vi "3 OCU.vi"(11 "MissionQueue":refnum<class "MissionQueue.lvclass">) -> ()   [LabVIEW 2011]
uses:
  2-RIO/2 Typedefs/setpoints to boat.ctl
  2-RIO/2 Typedefs/sail setpt.ctl
  2-RIO/2 Typedefs/rudder angle.ctl
  2-RIO/2 Typedefs/Velocity.ctl
  2-RIO/2 Typedefs/apparent wind direction.ctl
  2-RIO/2 Typedefs/apparent wind speed.ctl
  2-RIO/2 Typedefs/apparent wind.ctl
  2-RIO/2 Typedefs/heading.ctl
  2-RIO/2 Typedefs/UTM Location.ctl
  2-RIO/2 Typedefs/Which Boat.ctl
  2-RIO/2 Typedefs/generalized sensor status.ctl
  2-RIO/2 Typedefs/indicator LED.ctl
  2-RIO/2 Typedefs/generalized actuator status.ctl
  Classes/Missions/MissionQueue/MissionQueue.lvclass
  2x3-RIO-OCU Comm/2x3 Typedefs/missionTypes.ctl
  2-RIO/2 Typedefs/manual override.ctl
  2-RIO/2 Globals/2 Global.vi
  Classes/Missions/Drive/Drive.lvclass
panel:
  out "Override Rudder Angle":dbl(slide) scale=-30.0..30.0
  out "Override Sail Value":dbl(slide) scale=0.0..1.0
  in  "OVERRIDE?":bool
  in  "OCU Tab Control":T1(tab)
  out "Connected":bool
  in  "Connect":bool
  out "Rudder Actuator Status":T2
  out "Sail Actuator Status":T2
  out "Wind Sensor Status":T4
  out "Location Sensor Status":T4
  out "Direction Sensor Status":T4
  in  "Add Mission":bool
  in  "Load":bool
  in  "Load Mission":path
  in  "Mission Types":T5
  in  "Desired UTM\nLocation (Drive)":T6 caption="Desired UTM Location"
  in  "Distance \nThreshold (Drive)":dbl caption="Distance Threshold"
  in  "Globals":T7(tab)
  out "Which Boat Am I?":T8 items=["Small RC", "Large RC", "Final Boat", "Simulator"]
  in  "Battery Voltage":dbl
  out "Robot\nHeading":T9 format="%05.1f"
  out "Robot UTM Location":T6
  out "Robot Velocity":T10
  out "Overview Image":T11(plugin-control)
  out "Absolute Wind":T10
  out "Apparent Wind\nDirection":T12
  out "Apparent Wind\nSpeed":T13
  out "Apparent Wind":T14
  out "Current Destination":T6
  out "Setpoints to boat":T15
  out "Sail Position":T16
  out "Rudder Angle":T17
  # "Manual Overide Control"
  # "Full Out = RIGHT"
  # "Out = UP"
  # "In = DOWN"
  # "Full In = LEFT"
  # "PORT"
  # "STARB"
  # "A"
  # "G"
  # "S"
  # "<--"
  # "D"
  # "-->"
  # "F"
  # "should be a map here that you can clique on"
  # "logging..."
  # "As Measured"
  # "From Planning Functions"
  # "Path Planning"
  # "(this is not a cluster because subitems\nare generated in parallel code)"
  # "Mission Definition Stuff Goes HERE"
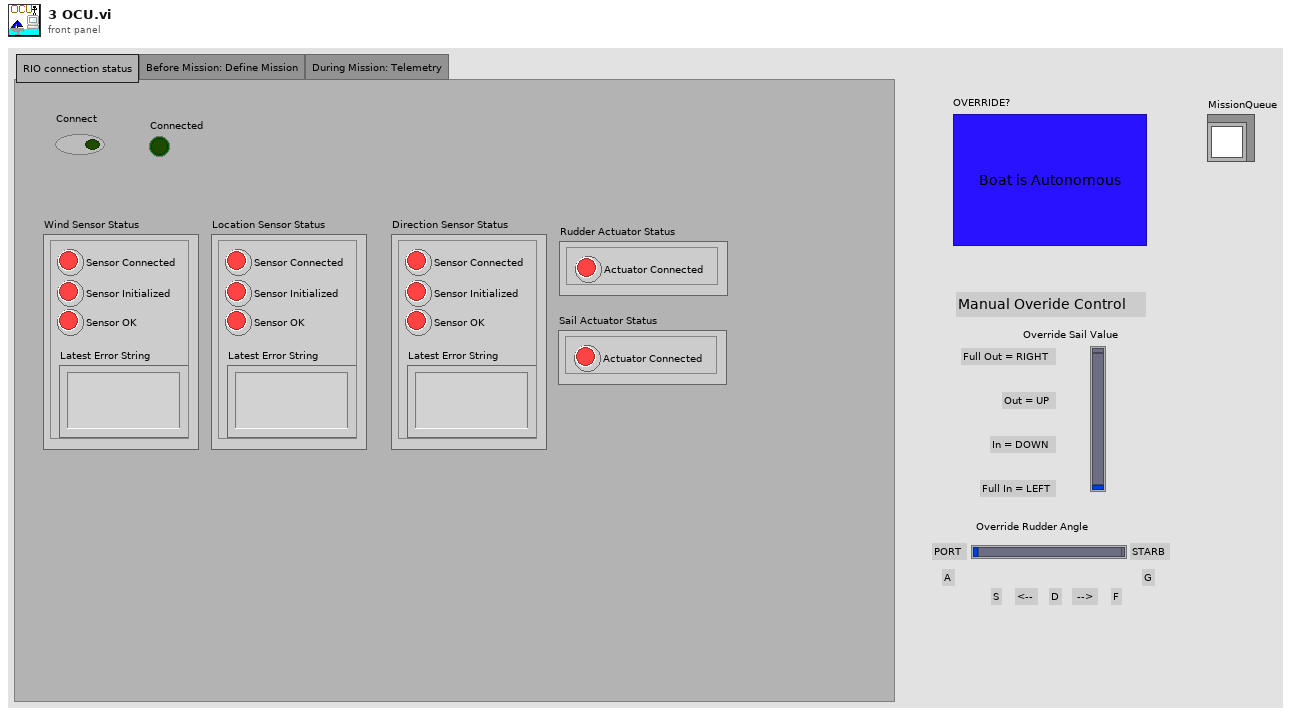
[diagram p1: front panel]
types:
  T1 = enum32{"RIO connection status", "Before Mission: Define Mission", "During Mission: Telemetry"}
  T2 = typedef "generalized actuator status.ctl" = cluster{"Actuator Connected":T3}
  T3 = typedef "indicator LED.ctl" = bool
  T4 = typedef "generalized sensor status.ctl" = cluster{"Sensor Connected":T3, "Sensor Initialized":T3, "Sensor OK":T3, "Latest Error String":string}
  T5 = typedef "missionTypes.ctl" = enum32{"Drive"}
  T6 = typedef "UTM Location.ctl" = cluster{"UTM Zone":dbl, "Hemisphere":enum16{"North", "South"}, "East":dbl, "North":dbl}
  T7 = enum32{"How Am I", "Where Am I", "What's Around Me", "Path Planning"}
  T8 = typedef "Which Boat.ctl" = u16
  T9 = typedef "heading.ctl" = dbl
  T10 = typedef "Velocity.ctl" = cluster{"East":dbl, "North":dbl}
  T11 = typedef "IMAQ Image.ctl" = refnum<image>
  T12 = typedef "apparent wind direction.ctl" = dbl
  T13 = typedef "apparent wind speed.ctl" = dbl
  T14 = typedef "apparent wind.ctl" = cluster{"Toward Fore":dbl, "Toward Starboard":dbl}
  T15 = typedef "setpoints to boat.ctl" = cluster{"Sail Position":T16, "Rudder Angle":T17}
  T16 = typedef "sail setpt.ctl" = dbl
  T17 = typedef "rudder angle.ctl" = dbl
  T18 = typedef "manual override.ctl" = cluster{"Override Active":bool, "Setpoints":T15}
  T19 = typedef "eventvkey.ctl" = enum16{"ASCII", "Enter", "Return", "Shift", "Ctrl", "Alt", "Cmd", "Opt", "Caps", "NumLock", "Clear", "Break", "Up", "Down", "Left", "Right", "Insert", "Delete", "Home", "End", "PageUp", "PageDown", "Escape", "Help", "Pause", "ScrollLock", "F1", "F2", "F3", "F4", "F5", "F6", "F7", "F8", "F9", "F10", "F11", "F12", "F13", "F14", "F15", "F16", "F17", "F18", "F19", "F20", "F21", "F22", "F23", "F24", "Play", "VolumeUp", "VolumeDown", "Mute", "Two Byte Char"}
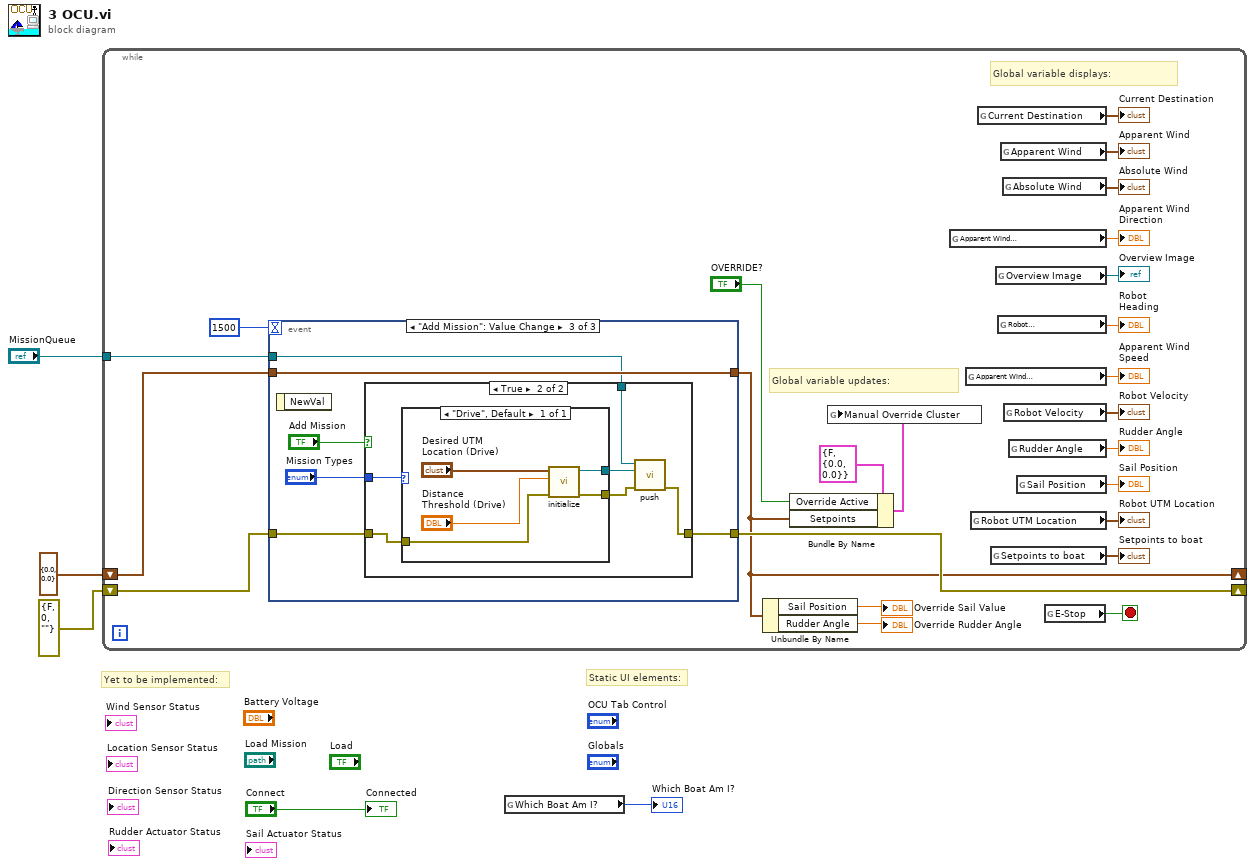
[diagram p0: block diagram]
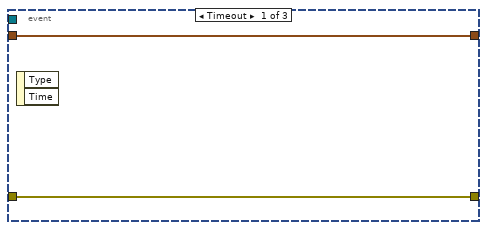
[diagram p2: hidden frame]
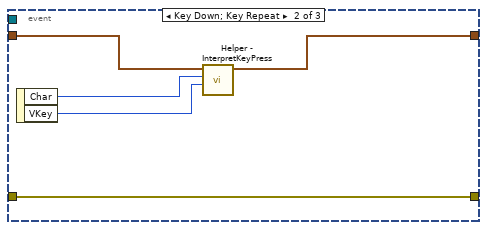
[diagram p3: hidden frame]
diagram:
  # "Static UI elements:"
  # "Yet to be implemented:"
  n1 = while {
    tunnel: "MissionQueue" -> [w6]
    shift-right: [w11] -> _
    shift-left: errorcluster {"status"=FALSE, "code"=0, "source"=""} ("error out") -> [w12]
    shift-right: [w9] -> _
    shift-left: T15 {"Sail Position"=0.0, "Rudder Angle"=0.0} ("Setpoints") -> [w16]
    stop <- w29 stop-if-true
    # "Global variable updates:"
    # "Global variable displays:"
    n2 = event shown="[2] \"Add Mission\": Value Change" {
      selector: _ -> [_ _ _]
      dyn-events: _ -> [_ _ _]
      timeout: 1500 -> [_ _ _]
      tunnel: w16 -> [w31 w36 w42]
      tunnel: [w31 w35 w42] -> w9
      tunnel: w12 -> [w30 w32 w39]
      tunnel: w6 -> [_ _ w40]
      tunnel: [w30 w32 w38] -> w11
      event Timeout {
        n3 = event-data() -> ()  [unwired: 1 in, 2 out]
      }
      event Key Down; Key Repeat {
        n4 = event-data() -> ("Char"=w34:i16, "VKey"=w33:T19)  [unwired: 1 in]
        n5 = call "Helper - InterpretKeyPress.vi"("VKey"=w33, "Char"=w34, "Command In"=w36) -> ("Command Out"=w35:T15)  [unwired: 8 in]
      }
      event "Add Mission": Value Change {
        n6 = event-data() -> ()  [unwired: 1 in, 1 out]
        n7 = case shown="True" "Add Mission" {
          tunnel: "Mission Types" -> [_ w49]
          tunnel: w40 -> [_ w48]
          tunnel: w39 -> [w43 w45]
          tunnel: [w43 w44] -> w38
          frame False {
          }
          frame True {
            n8 = case shown="\"Drive\", Default" w49 {
              tunnel: [w52] -> w47
              tunnel: [w51] -> w46
              tunnel: w45 -> [w50]
              frame "Drive", Default {
                n9 = call "initialize.vi"("error in (no error)"=w50, "Distance Threshold"="Distance \nThreshold (Drive)", "Desired UTM Location"="Desired UTM\nLocation (Drive)") -> ("error out"=w51:errorcluster, "Drive Mission"=w52:refnum<class "Drive.lvclass">)  [unwired: 7 in]
              }
            }
            n10 = call "push.vi"("error in (no error)"=w46, "Mission.lvclass"=w47, "MissionQueue in"=w48) -> ("error out"=w44:errorcluster)  [unwired: 7 in, 1 out]
          }
        }
      }
    }
    n11 = Unbundle By Name(w9) -> ("Sail Position"=→"Override Sail Value":T16, "Rudder Angle"=→"Override Rudder Angle":T17)
    n12 = Bundle By Name(cluster=T18 {"Override Active"=FALSE, "Setpoints"={"Sail Position"=0.0, "Rudder Angle"=0.0}} ("Manual Override Cluster"), "Override Active"="OVERRIDE?", "Setpoints"=w9) -> (w13:T18)
    n13 = global write "2 Global.vi" "Manual Override Cluster"(w13) -> ()
    n14 = global read "2 Global.vi" "Apparent Wind\nDirection"() -> (→"Apparent Wind\nDirection":T12)
    n15 = global read "2 Global.vi" "Apparent Wind\nSpeed"() -> (→"Apparent Wind\nSpeed":T13)
    n16 = global read "2 Global.vi" "Robot UTM Location"() -> (→"Robot UTM Location":T6)
    n17 = global read "2 Global.vi" "Current Destination"() -> (→"Current Destination":T6)
    n18 = global read "2 Global.vi" "Setpoints to boat"() -> (→"Setpoints to boat":T15)
    n19 = global read "2 Global.vi" "Overview Image"() -> (→"Overview Image":T11)
    n20 = global read "2 Global.vi" "Robot\nHeading"() -> (→"Robot\nHeading":T9)
    n21 = global read "2 Global.vi" "Apparent Wind"() -> (→"Apparent Wind":T14)
    n22 = global read "2 Global.vi" "Absolute Wind"() -> (→"Absolute Wind":T10)
    n23 = global read "2 Global.vi" "Robot Velocity"() -> (→"Robot Velocity":T10)
    n24 = global read "2 Global.vi" "Rudder Angle"() -> (→"Rudder Angle":T17)
    n25 = global read "2 Global.vi" "Sail Position"() -> (→"Sail Position":T16)
    n26 = global read "2 Global.vi" "E-Stop"() -> (w29:bool)
  }
  n27 = global read "2 Global.vi" "Which Boat Am I?"() -> (→"Which Boat Am I?":T8)
  "Connected" <- "Connect"
